vi "TurretAim_OperatorAssist.vi"(0 "TargetPos":dbl format="%#_13g", 2 "FullRight":bool, 3 "Start":bool, 4 "FullLeft":bool, 5 "TargetFound":bool, 6 "ManualOverride":bool, 7 "Reacquire":bool) -> (1 "TurretPos":dbl format="%#_13g")   [LabVIEW 2016]
panel:
  in  "TurretState":T1(ring)
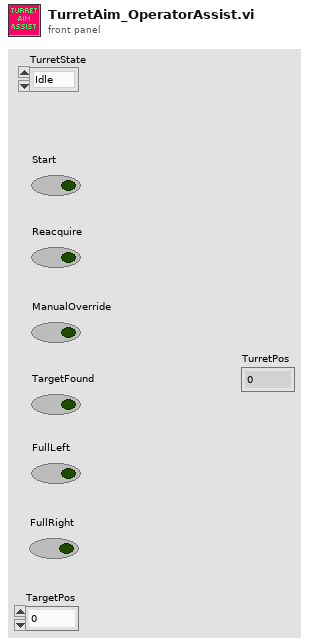
[diagram p1: front panel]
types:
  T1 = enum16{"Idle", "SearchLeft", "SearchRight", "FindNewTarget", "TargetAcquired"}
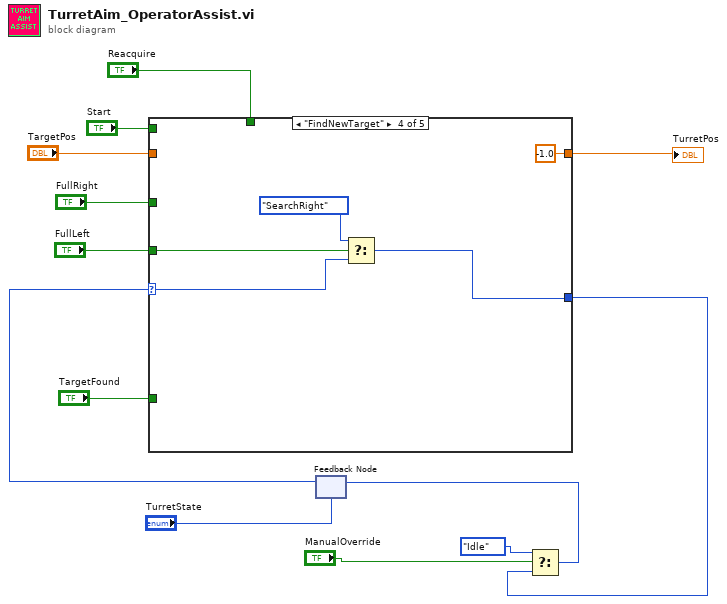
[diagram p0: block diagram]
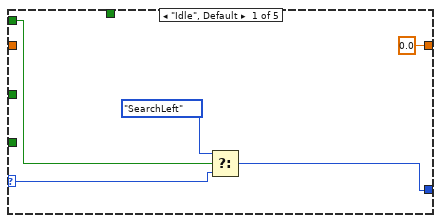
[diagram p2: hidden frame]
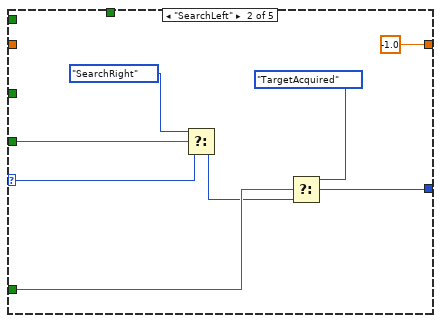
[diagram p3: hidden frame]
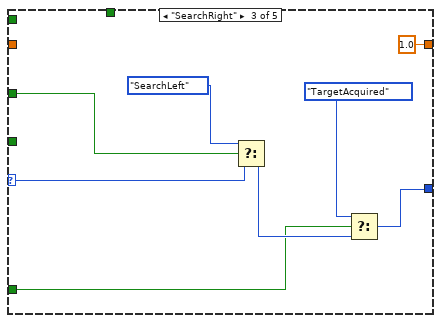
[diagram p4: hidden frame]
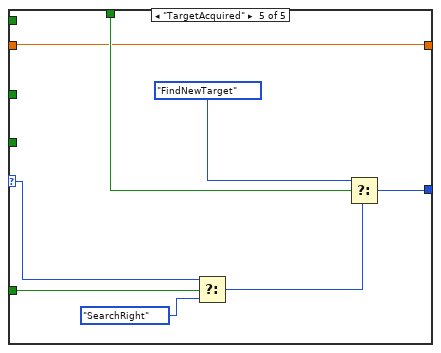
[diagram p5: hidden frame]
diagram:
  n1 = feedback #1("TurretState") -> (w13:T1)
  n2 = case shown="\"FindNewTarget\"" w13 {
    selector: w13 -> [w18 w26 w30 w38 w42]
    tunnel: "TargetFound" -> [_ w24 w31 _ w44]
    tunnel: "FullLeft" -> [_ w23 _ w39 _]
    tunnel: [w15 w21 w28 w36 w45] -> w5
    tunnel: "FullRight" -> [_ _ w32 _ _]
    tunnel: "Reacquire" -> [_ _ _ _ w47]
    tunnel: "Start" -> [w17 _ _ _ _]
    tunnel: [0.0 ("TargetPos") -1.0 ("TurretPos") 1.0 ("TurretPos") -1.0 ("TargetPos") w40] -> w2
    tunnel: "TargetPos" -> [_ _ _ _ w40]
    frame "Idle", Default {
      n3 = Select(t=T1."SearchLeft", s=w17, f=w18) -> (s? t:f=w15:T1)
    }
    frame "SearchLeft" {
      n4 = Select(t=T1."SearchRight", s=w23, f=w26) -> (s? t:f=w22:T1)
      n5 = Select(t=T1."TargetAcquired", s=w24, f=w22) -> (s? t:f=w21:T1)
    }
    frame "SearchRight" {
      n6 = Select(t=T1."SearchLeft", s=w32, f=w30) -> (s? t:f=w33:T1)
      n7 = Select(t=T1."TargetAcquired", s=w31, f=w33) -> (s? t:f=w28:T1)
    }
    frame "FindNewTarget" {
      n8 = Select(t=T1."SearchRight", s=w39, f=w38) -> (s? t:f=w36:T1)
    }
    frame "TargetAcquired" {
      n9 = Select(t=w42, s=w44, f=T1."SearchRight" ("t")) -> (s? t:f=w43:T1)
      n10 = Select(t=T1."FindNewTarget", s=w47, f=w43) -> (s? t:f=w45:T1)
    }
  }
  "TurretPos" <- w2
  n11 = Select(t=T1."Idle", s="ManualOverride", f=w5) -> (s? t:f=w3:T1)
  n12 = feedback-in #1(w3) -> ()
